vi "InfoPopUp.vi"(9 "Text to Match":string, 10 "Iteration Count":u64) -> ()   [LabVIEW 2015]
panel:
  out "Message":string
  # "Please click anywhere on this screen to close this window"
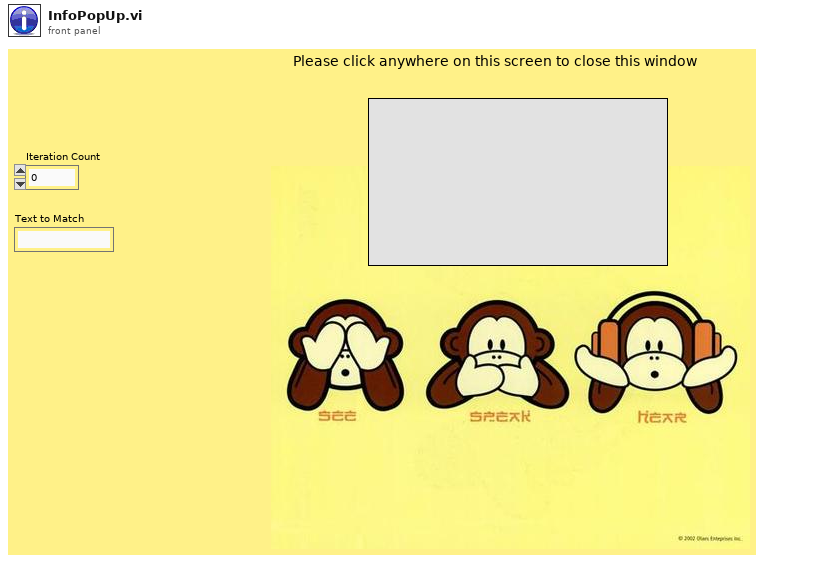
[diagram p1: front panel]
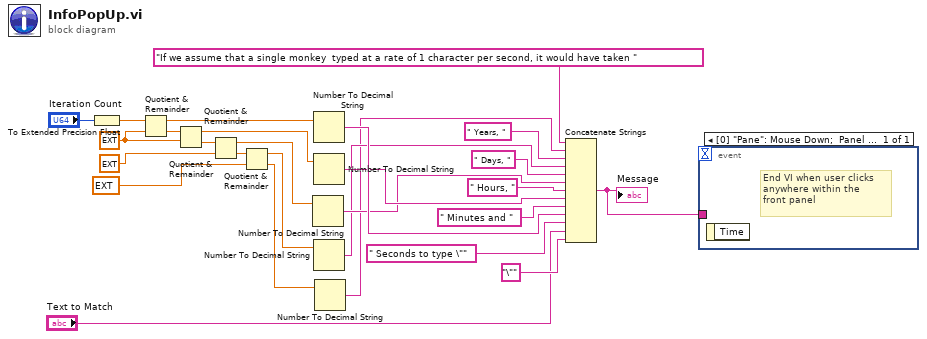
[diagram p0: block diagram]
diagram:
  w14 = ext 60.0 ("y")
  n1 = To Extended Precision Float(1:"Iteration Count") -> (0:w12:ext)
  n2 = Quotient & Remainder(x=w12, y=w14) -> (x-y*floor(x/y)=w15:ext, floor(x/y)=w11:ext)
  n3 = Quotient & Remainder(x=w11, y=w14) -> (x-y*floor(x/y)=w16:ext, floor(x/y)=w10:ext)
  n4 = Quotient & Remainder(x=w10, y=ext 24.0) -> (x-y*floor(x/y)=w17:ext, floor(x/y)=w7:ext)
  n5 = Quotient & Remainder(x=w7, y=ext 365.0) -> (x-y*floor(x/y)=w6:ext, floor(x/y)=w4:ext)
  n6 = Number To Decimal String(number=w17) -> (decimal integer string=w23:string)  [unwired: 1 in]
  n7 = Number To Decimal String(number=w15) -> (decimal integer string=w25:string)  [unwired: 1 in]
  n8 = Number To Decimal String(number=w16) -> (decimal integer string=w24:string)  [unwired: 1 in]
  n9 = Number To Decimal String(number=w6) -> (decimal integer string=w22:string)  [unwired: 1 in]
  n10 = Number To Decimal String(number=w4) -> (decimal integer string=w3:string)  [unwired: 1 in]
  n11 = Concatenate Strings("If we assume that a single monkey  typed at a rate of 1 character per second, it would have taken " ("string"), w3, " Years, " ("string"), w22, " Days, ", w23, " Hours, ", w24, " Minutes and ", w25, " Seconds to type \"", "Text to Match", "\"" ("string")) -> (w8:string)
  "Message" <- w8
  n12 = event shown="[0] \"Pane\": Mouse Down;  Panel Close" {
    selector: _ -> [_]
    dyn-events: _ -> [_]
    timeout: _ -> [_]
    tunnel: w8 -> [_]
    event Mouse Down; Panel Close {
      # "End VI when user clicks\nanywhere within the \nfront panel"
      n13 = event-data() -> ()  [unwired: 1 in, 1 out]
    }
  }
